vi "Periodic Tasks.vi"(8 "error in":errorcluster) -> ()   [LabVIEW 2018]
doc: "This VI runs in parallel to other tasks. It can contain as many user-defined periodic loops as you need. These can carry out PID or other sorts of timed response."
uses:
  <vilib>/Rock Robotics/WPI/Utilities/WPI_GetSetVariantRefNum.vi
  <vilib>/Rock Robotics/WPI/Ultrasonic/WPI_SonarSRF04DigitalRefNum Registry Get.vi
  <vilib>/Rock Robotics/Network Tables/NT Read Boolean.vi
  <vilib>/Rock Robotics/Network Tables/NT Write Boolean.vi
  <vilib>/Rock Robotics/WPI/Solenoid/Deprecated/WPI_SolenoidSetBool.vi
  <vilib>/Rock Robotics/WPI/Ultrasonic/WPI_SonarSRF04DigitalGetRange.vi
  <vilib>/Rock Robotics/Network Tables/NT Write Number.vi
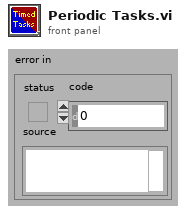
[diagram p1: front panel]
types:
  T1 = typedef "WPI_EncoderDevRef.ctl" = cluster{"DevStatus":errorcluster, "EncoderIndex":T2, "CounterIndex":T3, "DistancePerCount":dbl, "Decoding Type":T4}
  T2 = typedef "FPGA_EncoderIdx.ctl" = enum8{"Enc 0", "Enc 1", "Enc 2", "Enc 3", "Enc 4", "Enc 5", "Enc 6", "Enc 7", "Invalid"}
  T3 = typedef "FPGA_CounterCtrSystemIndex.ctl" = enum8{"Ctr 0", "Ctr 1", "Ctr 2", "Ctr 3", "Ctr 4", "Ctr 5", "Ctr 6", "Ctr 7", "Invalid"}
  T4 = typedef "WPI_EncoderType.ctl" = enum16{"1x", "2x", "4x"}
  T5 = typedef "WPI_JoystickDevRef.ctl" = cluster{"Device":T6}
  T6 = typedef "WPI_JoystickDeviceEnum.ctl" = enum16{"USB 0", "USB 1", "USB 2", "USB 3", "USB 4", "USB 5"}
  T7 = typedef "WPI_RobotDriveDevRef.ctl" = cluster{"DevStatus":errorcluster, "Motors[]":T8[], "Square Inputs":bool, "Max Output":dbl}
  T8 = typedef "WPI_MotorControlDeviceRef.ctl" = cluster{"DeviceStatus":errorcluster, "Type":T9, "PWM":cluster{"PWM Channel":T10, "DeadBand":T11}, "CAN":cluster{"Device Number":u8, "SetOutput VI Ref":variant, "GetOutput VI Ref":variant, "Enable VI Ref":variant, "Disable VI Ref":variant, "Data":variant}, "Invert":bool, "DIO PWM":cluster{"PWM \"Enable\" Channel":T10, "DIOChannel":T12, "PWM Rate":dbl}}
  T9 = typedef "WPI_MotorControlType.ctl" = enum16{"PWM", "CAN", "DIO PWM"}
  T10 = typedef "FPGA_DIOPWMChannel.ctl" = enum8{"PWM 0", "PWM 1", "PWM 2", "PWM 3", "PWM 4", "PWM 5", "PWM 6", "PWM 7", "PWM 8", "PWM 9", "PWM MXP 0", "PWM MXP 1", "PWM MXP 2", "PWM MXP 3", "PWM MXP 4", "PWM MXP 5", "PWM MXP 6", "PWM MXP 7", "PWM MXP 8", "PWM MXP 9", "Invalid"}
  T11 = typedef "WPI_PWMDeadband.ctl" = cluster{"Name":string, "maxPositivePwm":i32, "minPositivePwm":i32, "centerPwm":i32, "maxNegativePwm":i32, "minNegativePwm":i32, "angularRange":u16}
  T12 = typedef "FPGA_DIOChannel.ctl" = enum8{"DIO 0", "DIO 1", "DIO 2", "DIO 3", "DIO 4", "DIO 5", "DIO 6", "DIO 7", "DIO 8", "DIO 9", "DIO MXP 0", "DIO MXP 1", "DIO MXP 2", "DIO MXP 3", "DIO MXP 4", "DIO MXP 5", "DIO MXP 6", "DIO MXP 7", "DIO MXP 8", "DIO MXP 9", "DIO MXP 10", "DIO MXP 11", "DIO MXP 12", "DIO MXP 13", "DIO MXP 14", "DIO MXP 15", "SPI Port CS1", "SPI Port CS2", "SPI Port CS3", "SPI Port MISO", "SPI Port MOSI", "Invalid"}
  T13 = typedef "WPI_SolenoidDevRef.ctl" = cluster{"DevStatus":errorcluster, "Pneumatics Control Module":u8, "Forward Solenoid Channel":T14, "Reverse Solenoid Channel":T14}
  T14 = typedef "WPI_SolenoidChannel.ctl" = enum8{"Solenoid 0", "Solenoid 1", "Solenoid 2", "Solenoid 3", "Solenoid 4", "Solenoid 5", "Solenoid 6", "Solenoid 7", "Invalid"}
  T15 = typedef "WPI_UltrasonicDeviceRef.ctl" = cluster{"DevStatus":errorcluster, "Ping Channel":T12, "Echo Channel":T12, "CntIndex":T3}
  T16 = typedef "WPI_SwitchDevRef.ctl" = cluster{"DevStatus":errorcluster, "DIO Channel":T12, "CntIndex":T3, "Normally Closed":bool}
  T17 = cluster{"JoystickDevRef":T5, "RobotDriveDevRef":T7}
  T18 = typedef "WPI_CompressorDevRef.ctl" = cluster{"DevStatus":errorcluster, "Pneumatics Control Module":u8}
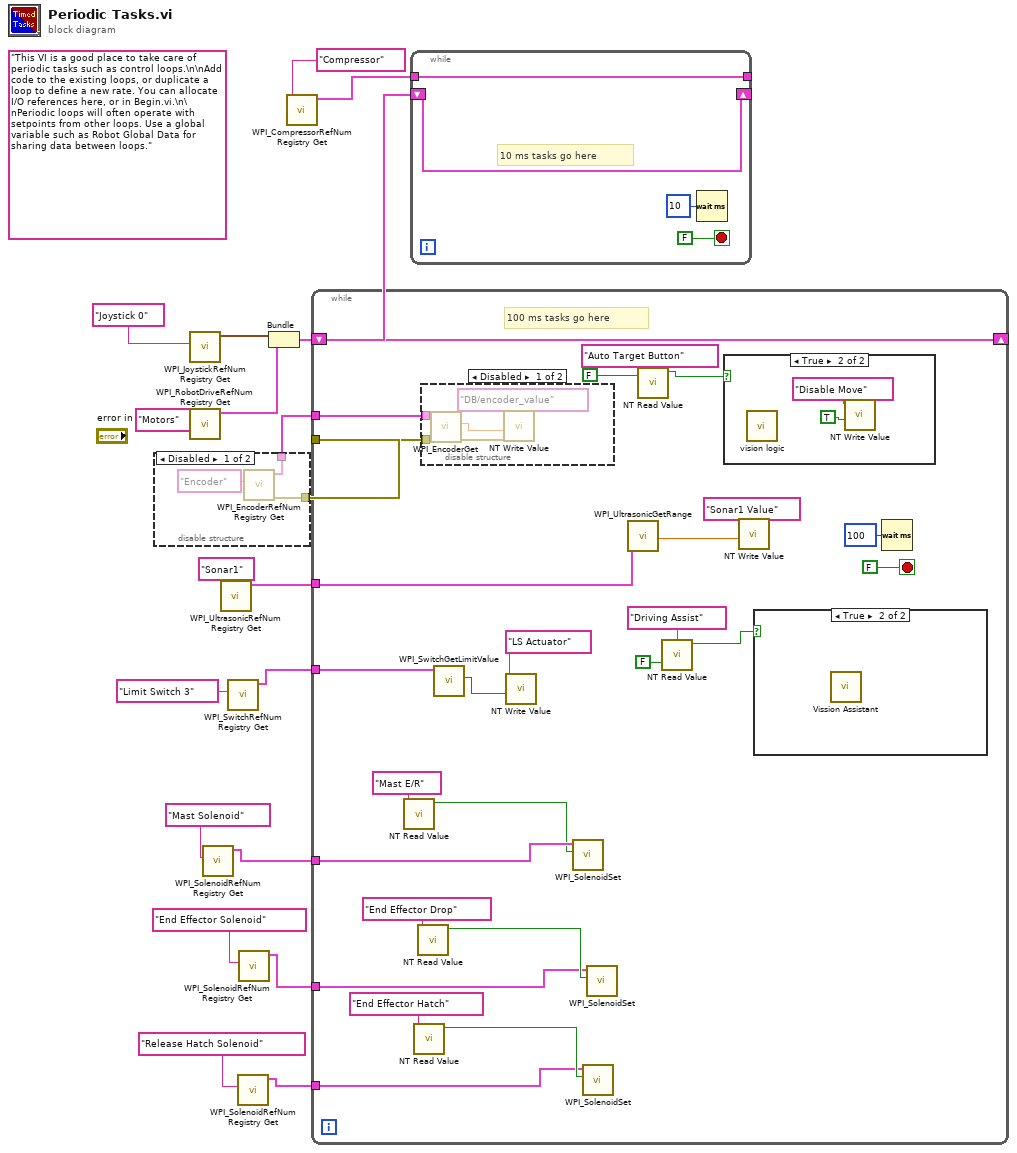
[diagram p0: block diagram]
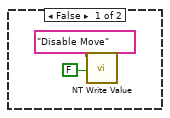
[diagram p4: hidden frame]
diagram:
  (unwired) "This VI is a good place to take care of periodic tasks such as control loops.\n\nAdd code to the existing loops, or duplicate a loop to define a new rate. You can allocate I/O references here, or in Begin.vi.\n\nPeriodic loops will often operate with setpoints from other loops. Use a global variable such as Robot Global Data for sharing data between loops."
  n1 = disable-structure shown="Disabled" {
    disable-tunnel: [w21 _] -> w14
    disable-tunnel: [w20 _] -> w13
    frame Disabled {
      n2 = call <vilib>:"WPI_EncoderRefNum Registry Get.vi"("refnum name"="Encoder") -> ("error out"=w20:errorcluster, "EncoderDevRef"=w21:T1)  [unwired: 9 in]
    }
    frame Enabled {
    }
  }
  n3 = call <vilib>:"WPI_JoystickRefNum Registry Get.vi"("refnum name"="Joystick 0") -> ("JoystickDevRef"=w17:T5)  [unwired: 1 in, 9 out]
  n4 = call <vilib>:"WPI_RobotDriveRefNum Registry Get.vi"("refnum name"="Motors") -> ("RobotDriveDevRef"=w16:T7)  [unwired: 1 in, 9 out]
  n5 = call <vilib>:"WPI_SolenoidRefNum Registry Get.vi"("refnum name"="Mast Solenoid") -> ("SolenoidDevRef"=w6:T13)  [unwired: 9 in, 1 out]
  n6 = call-poly <vilib>:"WPI_UltrasonicRefNum Registry Get.vi"("refnum name"="Sonar1") -> ("SonarSRF04DevRef"=w11:T15)  [unwired: 9 in, 1 out]
  n7 = call <vilib>:"WPI_SwitchRefNum Registry Get.vi"("refnum name"="Limit Switch 3") -> ("SwitchDevRef"=w9:T16)  [unwired: 9 in, 1 out]
  n8 = call <vilib>:"WPI_SolenoidRefNum Registry Get.vi"("refnum name"="Release Hatch Solenoid") -> ("SolenoidDevRef"=w1:T13)  [unwired: 9 in, 1 out]
  n9 = call <vilib>:"WPI_SolenoidRefNum Registry Get.vi"("refnum name"="End Effector Solenoid") -> ("SolenoidDevRef"=w3:T13)  [unwired: 9 in, 1 out]
  n10 = Bundle("JoystickDevRef"=w17, "RobotDriveDevRef"=w16) -> (w15:T17)  [unwired: 1 out]
  n11 = call <vilib>:"WPI_CompressorRefNum Registry Get.vi"("refnum name"="Compressor") -> ("CompressorDevRef"=w7:T18)  [unwired: 9 in, 1 out]
  n12 = while {
    shift-right: [w46] -> _
    shift-left: w15 -> [w46]
    tunnel: w14 -> [w45]
    tunnel: w13 -> [w44]
    tunnel: w11 -> [w43]
    tunnel: w9 -> [w37]
    tunnel: w6 -> [w30]
    tunnel: w3 -> [w24]
    tunnel: w1 -> [w23]
    stop <- FALSE stop-if-true
    # "100 ms tasks go here"
    n13 = call-poly <vilib>:"NT Read Value.vi"("Name"="Mast E/R") -> ("Boolean"=w29:bool)  [unwired: 9 in, 1 out]
    n14 = call-poly <vilib>:"NT Read Value.vi"("Name"="End Effector Hatch") -> ("Boolean"=w25:bool)  [unwired: 9 in, 1 out]
    n15 = call-poly <vilib>:"NT Read Value.vi"("Name"="End Effector Drop") -> ("Boolean"=w27:bool)  [unwired: 9 in, 1 out]
    n16 = disable-structure shown="Disabled" {
      disable-tunnel: w45 -> [w57 _]
      disable-tunnel: w44 -> [w53 _]
      frame Disabled {
        n17 = call <vilib>:"WPI_EncoderGet.vi"("error in (no error)"=w53, "EncoderDevRef"=w57) -> ("error out"=w54:errorcluster, "Distance"=w56:dbl)  [unwired: 4 in, 4 out]
        n18 = call-poly <vilib>:"NT Write Value.vi"("error in"=w54, "Numeric"=w56, "Name"="DB/encoder_value") -> ()  [unwired: 8 in, 1 out]
      }
      frame Enabled {
      }
    }
    n19 = call <vilib>:"WPI_SwitchGetLimitValue.vi"("SwitchDevRef"=w37) -> ("Switch Pressed"=w36:bool)  [unwired: 8 in, 2 out]
    n20 = call-poly <vilib>:"NT Write Value.vi"("Boolean"=w36, "Name"="LS Actuator") -> ()  [unwired: 9 in, 1 out]
    n21 = call-poly <vilib>:"WPI_SolenoidSet.vi"("Value"=w29, "SolenoidDevRef"=w30) -> ()  [unwired: 8 in, 2 out]
    n22 = call-poly <vilib>:"WPI_SolenoidSet.vi"("Value"=w25, "SolenoidDevRef"=w23) -> ()  [unwired: 8 in, 2 out]
    n23 = call-poly <vilib>:"WPI_SolenoidSet.vi"("Value"=w27, "SolenoidDevRef"=w24) -> ()  [unwired: 8 in, 2 out]
    n24 = call-poly <vilib>:"WPI_UltrasonicGetRange.vi"("SonarSRF04DevRef"=w43) -> ("Distance"=w42:dbl)  [unwired: 8 in, 2 out]
    n25 = call-poly <vilib>:"NT Read Value.vi"("Default Value"=FALSE, "Name"="Auto Target Button") -> ("Boolean"=w39:bool)  [unwired: 8 in, 1 out]
    n26 = call-poly <vilib>:"NT Read Value.vi"("Default Value"=FALSE, "Name"="Driving Assist") -> ("Boolean"=w32:bool)  [unwired: 8 in, 1 out]
    n27 = case shown="True" w39 {
      frame False {
        n28 = call-poly <vilib>:"NT Write Value.vi"("Boolean"=FALSE, "Name"="Disable Move") -> ()  [unwired: 9 in, 1 out]
      }
      frame True {
        n29 = call "vision logic.vi"() -> ()  [unwired: 16 in]
        n30 = call-poly <vilib>:"NT Write Value.vi"("Boolean"=TRUE, "Name"="Disable Move") -> ()  [unwired: 9 in, 1 out]
      }
    }
    n31 = call-poly <vilib>:"NT Write Value.vi"("Numeric"=w42, "Name"="Sonar1 Value") -> ()  [unwired: 9 in, 1 out]
    n32 = case shown="True" w32 {
      frame False {
      }
      frame True {
        n33 = call "Vission Assistant.vi"() -> ()  [unwired: 12 in]
      }
    }
    n34 = Wait (ms)(milliseconds to wait=u32 100) -> ()  [unwired: 1 out]
  }
  n35 = while {
    shift-right: [w59] -> _
    shift-left: w15 -> [w59]
    tunnel: w7 -> [w58]
    tunnel: [w58] -> _
    stop <- FALSE stop-if-true
    # "10 ms tasks go here"
    n36 = Wait (ms)(milliseconds to wait=u32 10) -> ()  [unwired: 1 out]
  }
